vi "MS_Var_to_Comm_Analog.vi"(11 "Boolean":bool) -> (1 "values":T1[](array[typedef]) {"value" format="%#_15f"})   [LabVIEW 2016, in "DNP3_Master_Station_Template.lvlib"]
uses:
  DNP3_Master_Station_Template.lvlib
  <vilib>/DNP3/DNP3_Master/Analog Info.ctl
  <vilib>/Utility/file.llb/Read Delimited Spreadsheet (string).vi
  <vilib>/DNP3/DNP3_Master.lvlib
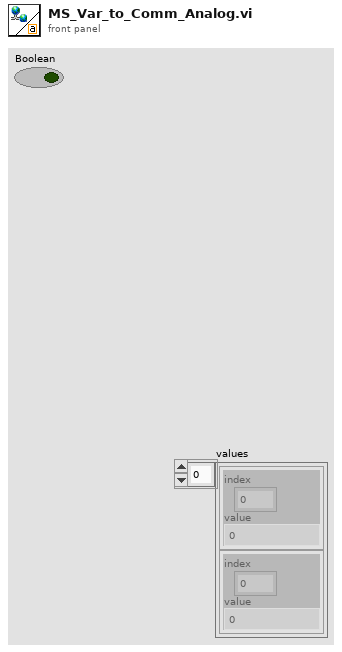
[diagram p1: front panel]
types:
  T1 = typedef "DNP3_Master.lvlib/Analog Info.ctl" = cluster{"index":u16, "value":dbl}
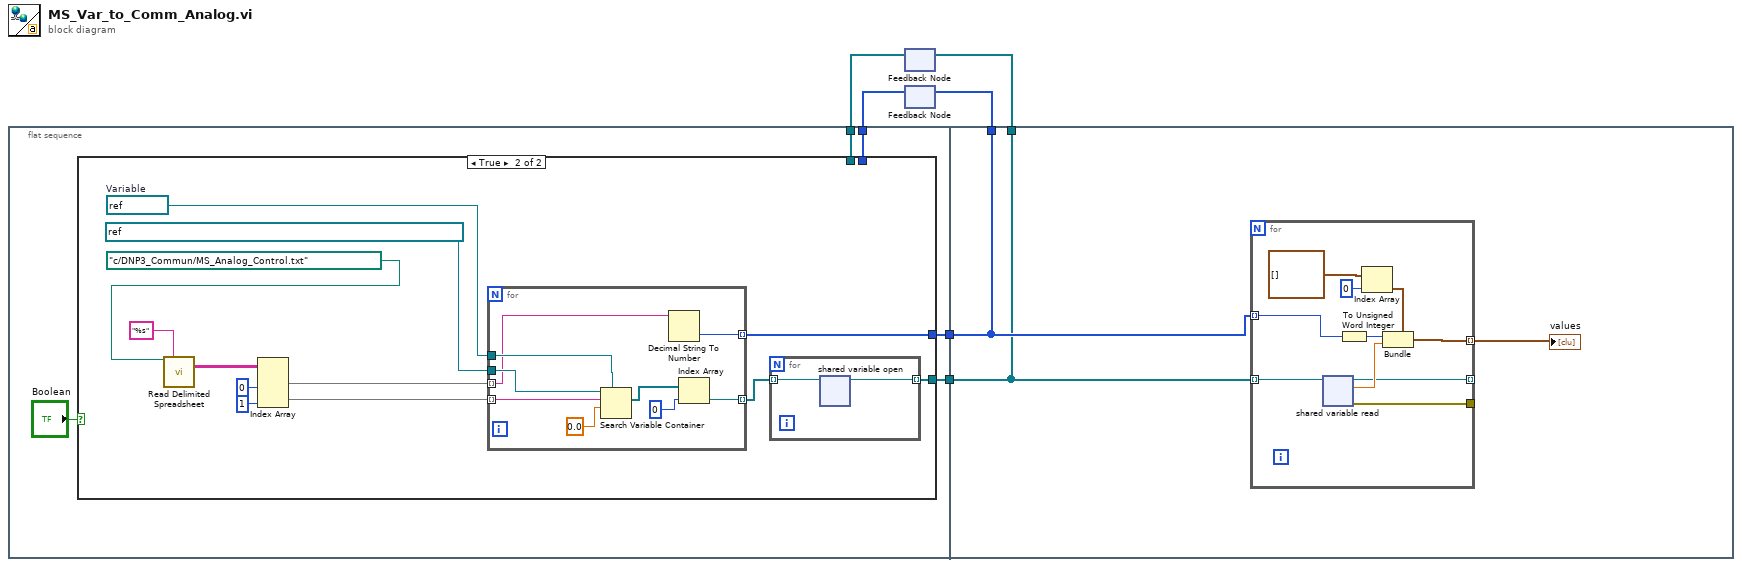
[diagram p0: block diagram]
diagram:
  n1 = flat-sequence {
    tunnel: [w11] -> w6
    tunnel: [w9] -> w5
    tunnel: w3 -> [w8]
    tunnel: w1 -> [w7]
    tunnel: w6 -> [w37]
    tunnel: w5 -> [w38]
    tunnel: [w38] -> w4
    tunnel: [w37] -> w2
    frame #0 {
      n2 = case shown="True" "Boolean" {
        tunnel: [w12 w14] -> w11
        tunnel: [w13 w16] -> w9
        tunnel: w8 -> [w13 _]
        tunnel: w7 -> [w12 _]
        frame False {
        }
        frame True {
          w18 = refnum<k21> refnum  # Variable
          n3 = call-poly <vilib>:"Read Delimited Spreadsheet.vi"("file path (dialog if empty)"=path "c:/DNP3_Commun/MS_Analog_Control.txt" ("file path (use dialog)"), "format (%s)"="%s") -> ("all rows"=w22:string[][])  [unwired: 8 in, 5 out]
          n4 = Index Array(array=w22, index (col) #1=0 ("disabled index (col)"), index (col) #2=1 ("index (col)")) -> (element #1=w17:string[], element #2=w25:string[])  [unwired: 2 in]
          n5 = for {
            tunnel: w18 -> [w34]
            tunnel: refnum<k21> "ni.var.psp://localhost/MS_Data_Variables/MS_Analog_Control/" ("container refnum in") -> [w33]
            tunnel: w17 -> [w29] mode=indexing
            tunnel: w25 -> [w32] mode=indexing
            tunnel: [w31] -> w15 mode=indexing
            tunnel: [w28] -> w16 mode=indexing
            n6 = Search Variable Container(7:w34, 9:0.0, 10:w32, 11:w33) -> (2:w36:refnum<k21>[])  [unwired: 2 in, 2 out]
            n7 = Decimal String To Number(string=w29) -> (number=w28:i32)  [unwired: 2 in, 1 out]
            n8 = Index Array(array=w36, index=0) -> (element=w31:refnum<k21>)
          }
          n9 = for {
            tunnel: w15 -> [w27] mode=indexing
            tunnel: [w26] -> w14 mode=indexing
            n10 = shared-variable-open(w27) -> (w26:refnum<k21>)  [unwired: 2 in, 1 out]
          }
        }
      }
    }
    frame #1 {
      n11 = for {
        tunnel: [w48] -> _
        tunnel: [w47] -> w39 mode=indexing
        tunnel: w37 -> [w46] mode=indexing
        tunnel: [w45] -> _ mode=indexing
        tunnel: w38 -> [w40] mode=indexing
        n12 = shared-variable-read(w46) -> (w45:refnum<k21>, w48:errorcluster, w49:dbl)  [unwired: 1 in, 1 out]
        n13 = To Unsigned Word Integer(number=w40) -> (unsigned 16bit integer=w41:u16)
        n14 = Index Array(array=T1[] [] ("values"), index=0) -> (element=w42:T1)
        n15 = Bundle(cluster=w42, "index"=w41, "value"=w49) -> (w47:T1)
      }
      "values" <- w39
    }
  }
  n16 = feedback #1() -> (w1:refnum<k21>[])  [unwired: 1 in]
  n17 = feedback-in #1(w2) -> ()
  n18 = feedback-in #2(w4) -> ()
  n19 = feedback #2() -> (w3:i32[])  [unwired: 1 in]
